vi "Append Linear Motion (Max Speed and Max Accel).vi"(8 "error in (no error)":errorcluster, 10 "Distance (in)":dbl, 11 "Motion Profile Generator in":refnum<class "Motion Profile Generator.lvclass">) -> (0 "error out":errorcluster, 3 "Motion Profile Generator out":refnum<class "Motion Profile Generator.lvclass">)   [LabVIEW 2019, in "Motion Profile Generator.lvclass"]
uses:
  Motion Profile Generator.lvclass
  Motion Profile Generator.lvclass/Motion Profile Generator.ctl
  Type Defs/Ramp - Velocity and Acceleration Mode.ctl
  Type Defs/Ramp - Final Snapshot Request.ctl
panel:
  in  "Final Velocity (in/s)":dbl
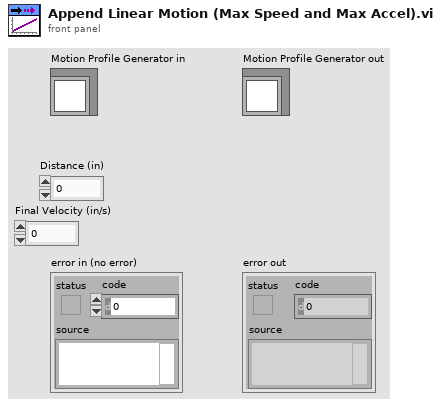
[diagram p1: front panel]
types:
  T1 = typedef "Motion Profile Generator.lvclass/Ramp - Final Snapshot Request.ctl" = enum16{"Movement Duration", "Distance"}
  T2 = typedef "Motion Profile Generator.lvclass/Ramp - Velocity and Acceleration Mode.ctl" = enum16{"Specific Acceleration", "Rampup and Rampdown Times"}
  T3 = typedef "Motion Profile Generator.lvclass/Control Boundaries.ctl" = cluster{"Max Speed (in/s)":dbl, "Max Acceleration (in/s2)":dbl, "Max Deceleration (in/s2)":dbl}
  T4 = typedef "Motion Profile Generator.lvclass/Motion Snapshot.ctl" = cluster{"Position (in)":dbl, "Velocity (in/s)":dbl, "Acceleration (in/s2)":dbl}
  T5 = typedef "Motion Profile Generator.lvclass/Motion Profile Point.ctl" = cluster{"Position (in)":dbl, "Velocity (in/s)":dbl, "Duration (ms)":dbl}
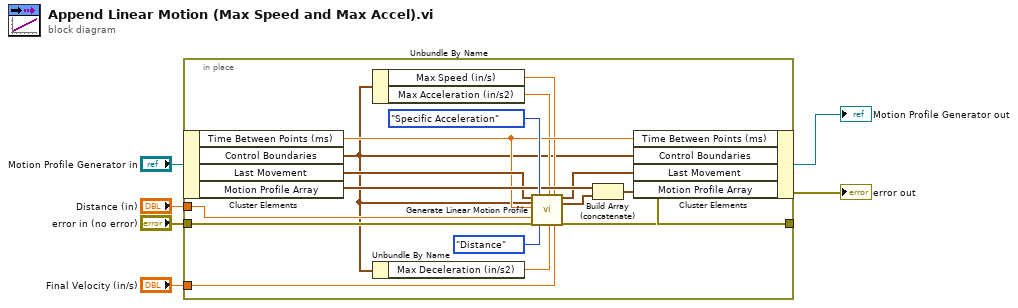
[diagram p0: block diagram]
diagram:
  n1 = in-place {
    in-place-border: "error in (no error)" -> [w20]
    in-place-border: [w19] -> w2
    in-place-border: "Distance (in)" -> [w12]
    in-place-border: "Final Velocity (in/s)" -> [w11]
    n2 = in-place-cluster #1("Motion Profile Generator in") -> ("Time Between Points (ms)"=w13:dbl, "Control Boundaries"=w8:T3, "Last Movement"=w15:T4, "Motion Profile Array"=w17:T5[])
    n3 = Unbundle By Name(w8) -> ("Max Speed (in/s)"=w10:dbl, "Max Acceleration (in/s2)"=w9:dbl)
    n4 = Unbundle By Name(w8) -> ("Max Deceleration (in/s2)"=w7:dbl)
    n5 = call "Generate Linear Motion Profile.vi"("Initial Snapshot"=w15, "Control Boundaries"=w8, "Time Between Points (ms)"=w13, "Distance (in)"=w12, "Error In"=w20, "Ramp - Velocity and Acceleration Mode"=Ramp_-_Velocity_and_Acceleration_Mode."Specific Acceleration", "Ramp - Final Snapshot Request"=Ramp_-_Final_Snapshot_Request."Distance", "Acceleration (in/s2)"=w9, "Deceleration (in/s2)"=w7, "Cruise Velocity (in/s)"=w10, "Final Velocity (in/s)"=w11) -> ("Final Snapshot"=w14:T4, "Motion Profile Portion"=w16:T5[], "Error Out"=w19:errorcluster)  [unwired: 6 in]
    n6 = Build Array (concatenate)(w17, w16) -> (w18:T5[])
    n7 = in-place-cluster #1("Time Between Points (ms)"=w13, "Control Boundaries"=w8, "Last Movement"=w14, "Motion Profile Array"=w18) -> (→"Motion Profile Generator out":refnum<class "Motion Profile Generator.lvclass">)
  }
  "error out" <- w2
